vi "Player Info.vi"(11 "Line Dancer in":refnum<class "Line Dancer.lvclass">) -> (1 "Victory Speech":string, 2 "Name":string, 3 "Line Dancer out":refnum<class "Line Dancer.lvclass">)   [LabVIEW 2015, in "Line Dancer.lvclass"]
uses:
  Line Dancer.lvclass
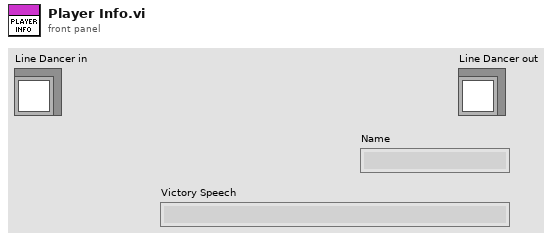
[diagram p1: front panel]
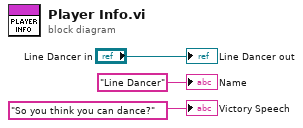
[diagram p0: block diagram]
diagram:
  "Line Dancer out" <- "Line Dancer in"
  "Name" <- "Line Dancer" ("Name")
  "Victory Speech" <- "So you think you can dance?" ("Victory Speech")
